vi "Set Grating.vi"(7 "Numeric":i32=75, 8 "error in (no error)":errorcluster, 11 "VISA resource name":refnum<visa-resource-name>) -> (0 "error out":errorcluster, 2 "Connected? 2":bool, 3 "VISA resource name out":refnum<visa-resource-name>)   [LabVIEW 2018]
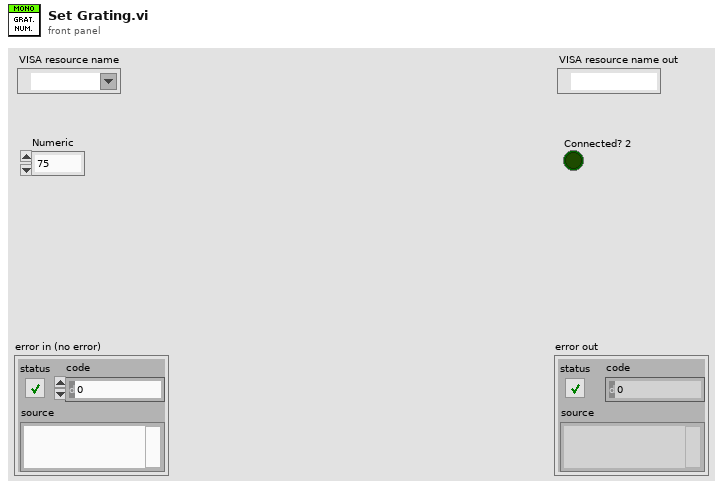
[diagram p1: front panel]
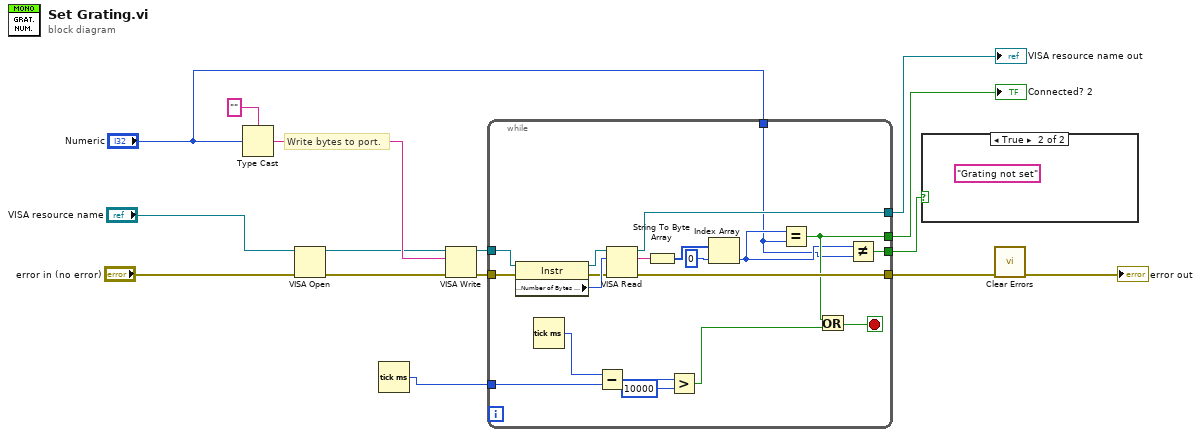
[diagram p0: block diagram]
diagram:
  # "Write bytes to port."
  n1 = Type Cast(type="", x="Numeric") -> (*(type *) &x=w11:string)
  n2 = VISA Open(error in (no error)="error in (no error)", VISA resource name="VISA resource name") -> (VISA resource name=w10:refnum<visa-resource-name>, error out=w9:errorcluster)  [unwired: 3 in]
  n3 = Tick Count (ms)() -> (millisecond timer value=w1:u32)
  n4 = VISA Write(VISA resource name=w10, write buffer=w11, error in (no error)=w9) -> (VISA resource name out=w12:refnum<visa-resource-name>, error out=w13:errorcluster)  [unwired: 1 out]
  n5 = while {
    tunnel: w12 -> [w29]
    tunnel: w13 -> [w30]
    tunnel: [w32] -> w4
    tunnel: [w31] -> w5
    tunnel: [w25] -> w14
    tunnel: [w23] -> w15
    tunnel: "Numeric" -> [w22]
    tunnel: w1 -> [w20]
    stop <- w17 stop-if-true
    n6 = property class="Instr"(reference=w29, error in=w30) -> (reference out=w28:refnum<visa-resource-name>, error out=w26:errorcluster, "Serial Settings:Number of Bytes at Serial Port"=w27:u32)
    n7 = Tick Count (ms)() -> (millisecond timer value=w21:u32)
    n8 = Subtract(x=w21, y=w20) -> (x-y=w19:u32)
    n9 = VISA Read(VISA resource name=w28, byte count=w27, error in (no error)=w26) -> (VISA resource name out=w32:refnum<visa-resource-name>, read buffer=w35:string, error out=w31:errorcluster)  [unwired: 1 out]
    n10 = String To Byte Array(string=w35) -> (unsigned byte array=w34:u8[])
    n11 = Greater?(x=w19, y=u32 10000) -> (0:w16:bool)
    n12 = Index Array(array=w34, index=0) -> (element=w24:u8)
    n13 = Equal?(x=w24, y=w22) -> (x = y?=w25:bool)
    n14 = Or(x=w25, y=w16) -> (x .or. y?=w17:bool)
    n15 = Not Equal?(x=w24, y=w22) -> (x != y?=w23:bool)
  }
  "Connected? 2" <- w14
  "VISA resource name out" <- w4
  n16 = case shown="True" w15 {
    frame False {
    }
    frame True {
      (unwired) "Grating not set"
    }
  }
  n17 = call <vilib>:"Clear Errors.vi"("error in (no error)"=w5) -> ("error out"=→"error out":errorcluster)  [unwired: 5 in, 1 out]
